vi "Inline Read.vi"(8 "error in (no error)":errorcluster, 9 "default values":variant[](array[variant]), 10 "keys":string[](array[string]), 11 "uData in":refnum<class "uData.lvclass">) -> (0 "error out":errorcluster, 1 "values":variant[](array[variant]), 3 "uData out":refnum<class "uData.lvclass">, 4 "found?":bool[](array[boolean]))   [LabVIEW 2023, in "uLib.lvlib" / "uData.lvclass"]
doc: "Dynamic dispatch method to perform an inline read operation.\n\n<B>THE \"INLINE\" DYNAMIC DISPATCH METHOD GROUP ARE THE ONLY METHODS THAT ARE ALLOWED TO ACCESS THE OBJECT PRIVATE DATA.</B>\n\nCONVERTED TO INLINE STATIC DISPATCH TO MITIGATE THE PERFORMANCE OVERHEAT HIT REALIZED IN INTIAL TESTING."
uses:
  uData.lvclass
  uData.lvclass/uData.ctl
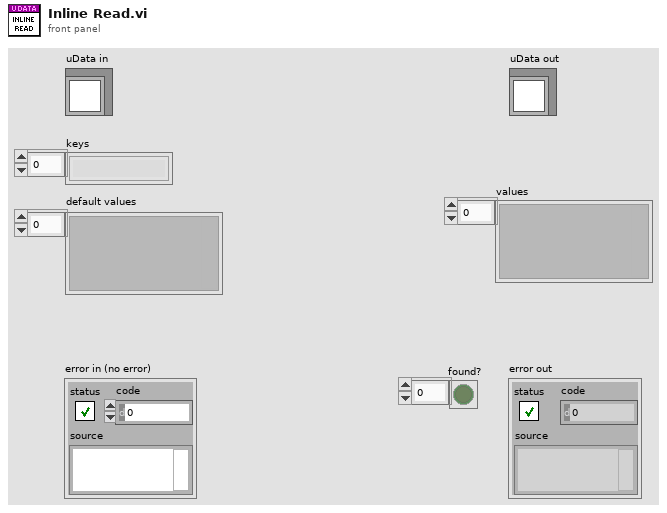
[diagram p1: front panel]
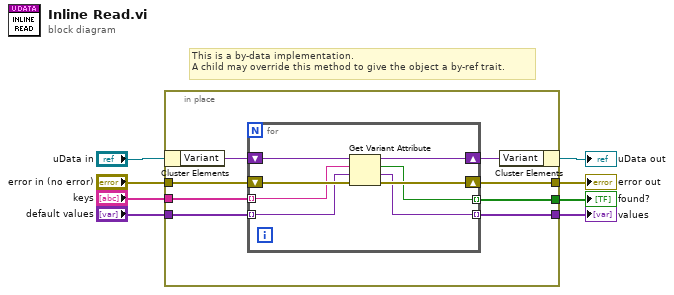
[diagram p0: block diagram]
diagram:
  # "This is a by-data implementation.\nA child may override this method to give the object a by-ref trait."
  n1 = in-place {
    in-place-border: [w14] -> w3
    in-place-border: "error in (no error)" -> [w13]
    in-place-border: [w12] -> w8
    in-place-border: "keys" -> [w9]
    in-place-border: "default values" -> [w11]
    in-place-border: [w10] -> w5
    n2 = in-place-cluster #1("uData in") -> ("Variant"=w16:variant)
    n3 = for {
      tunnel: [w20] -> w12 mode=indexing
      tunnel: w11 -> [w19] mode=indexing
      tunnel: [w18] -> w10 mode=indexing
      tunnel: w9 -> [w17] mode=indexing
      shift-right: [w23] -> w15
      shift-left: w16 -> [w24]
      shift-right: [w22] -> w14
      shift-left: w13 -> [w21]
      n4 = Get Variant Attribute(Variant=w24, name=w17, default value (empty Variant)=w19, error in=w21) -> (duplicate Variant=w23:variant, found=w20:bool, value=w18:variant, error out=w22:errorcluster)
    }
    n5 = in-place-cluster #1("Variant"=w15) -> (→"uData out":refnum<class "uData.lvclass">)
  }
  "error out" <- w3
  "found?" <- w8
  "values" <- w5
